vi "task2.vi"(6 "Zatrzymaj program":bool, 7 "Czy trójkąt jest prostokątny":bool, 8 "Oblicz":bool, 9 "Bok a":dbl(slide)=2.0 scale=0.0..10.0, 10 "Bok b":dbl(slide)=2.0 scale=0.0..10.0, 11 "Bok c":dbl(slide)=2.0 scale=0.0..10.0) -> (1 "Trójkąt:":string, 2 "Obwód trójkąta":dbl, 3 "Pole trójkąta":dbl)   [LabVIEW 2021]
doc: "Aplikacja na bazie maszyny stanów, która liczy pole i obwód podanego trójkąta. Użyty jest w nim program z wcześniejszego zadania. Program sprawdza czy podany trójkąt jest trójkątem prostokątnym."
panel:
  # "Podaj wielkość trójkąta:"
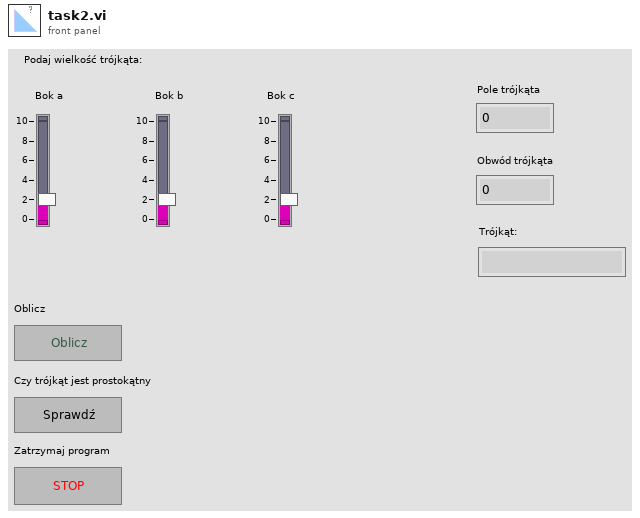
[diagram p1: front panel]
types:
  T1 = enum16{"Idle", "Czy prostokątny", "Oblicz", "Stop"}
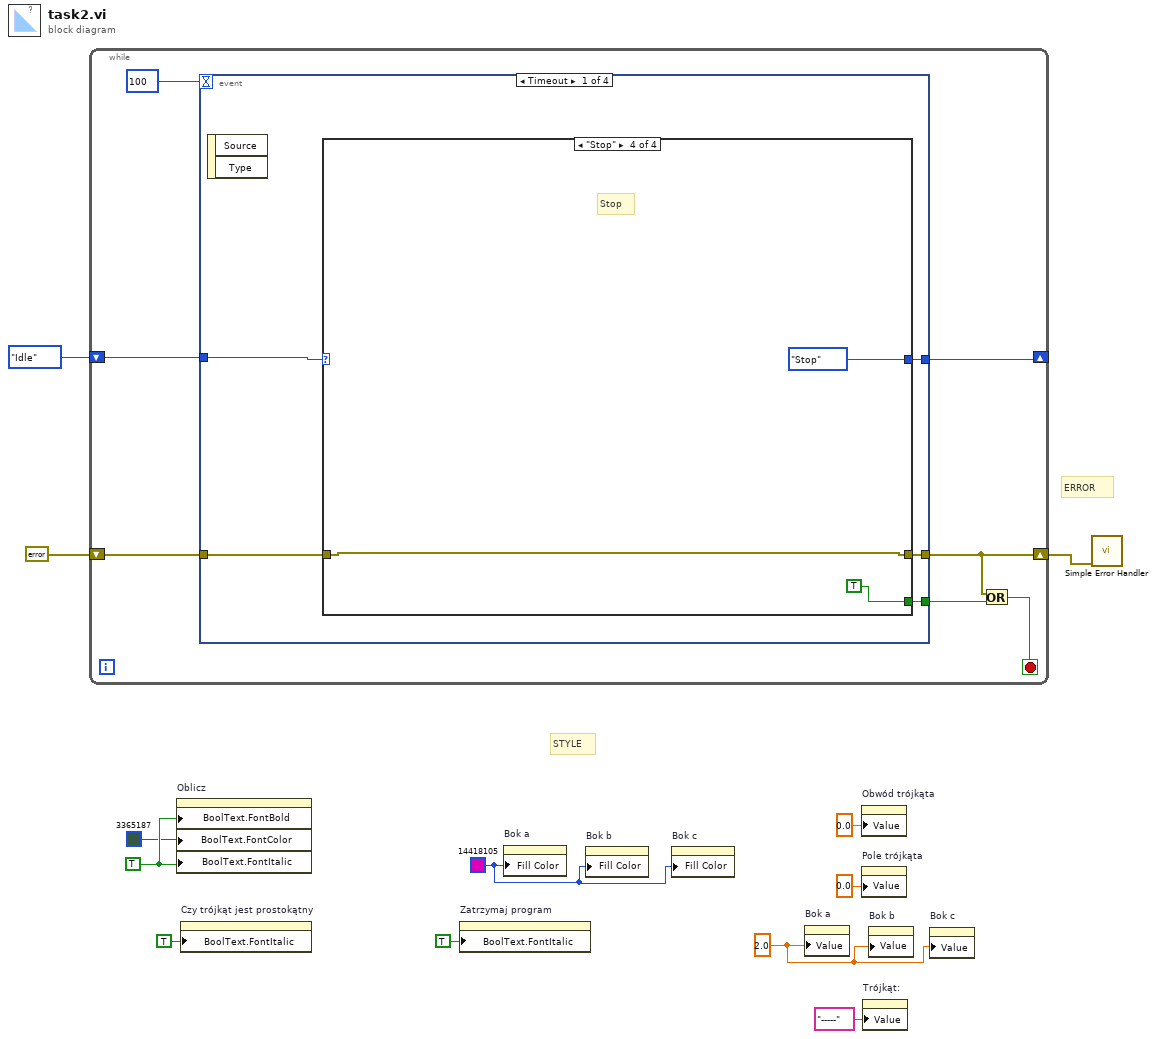
[diagram p0: block diagram]
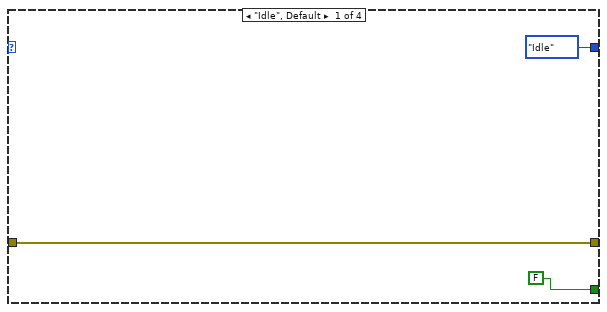
[diagram p2: hidden frame]
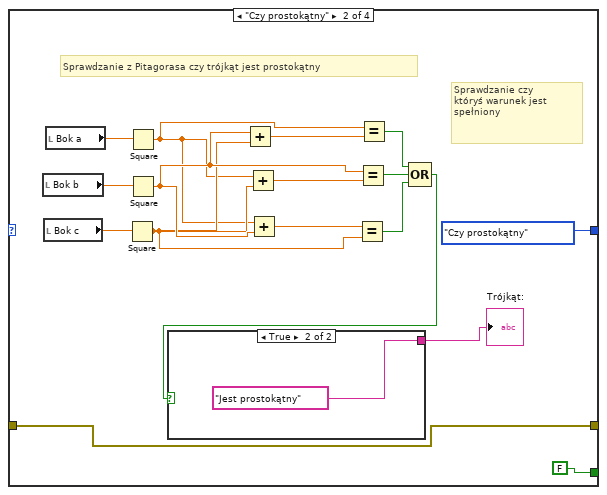
[diagram p3: hidden frame]
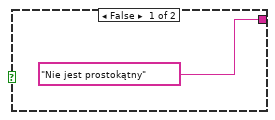
[diagram p4: hidden frame]
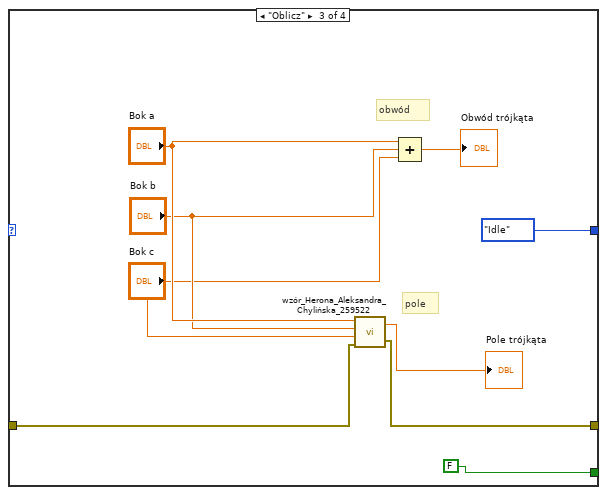
[diagram p5: hidden frame]
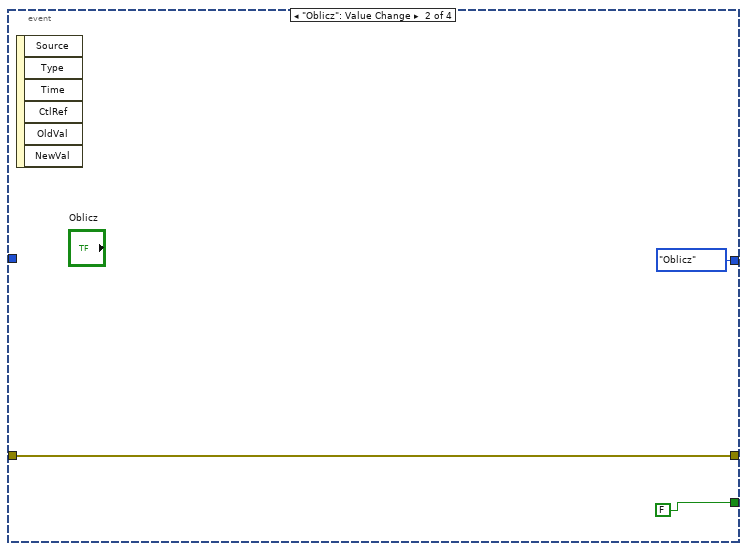
[diagram p6: hidden frame]
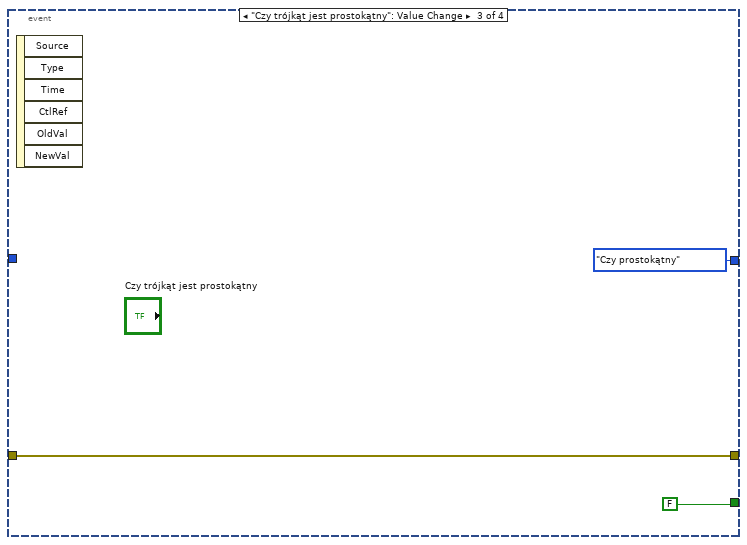
[diagram p7: hidden frame]
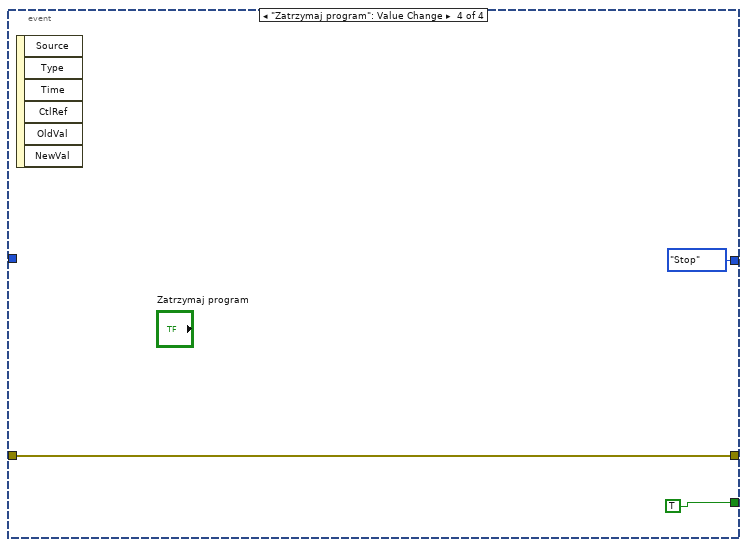
[diagram p8: hidden frame]
diagram:
  w4 = 2.0 ("Bok a")
  w8 = TRUE ("Boolean Text.Font:Italic")
  w9 = u32 14418105 ("Fill Color")
  # "ERROR"
  # "STYLE"
  n1 = while {
    shift-right: [w18] -> _
    shift-left: T1."Idle" -> [w19]
    shift-right: [w14] -> w10
    shift-left: errorcluster {"status"=FALSE, "code"=0, "source"=""} ("error in (no error)") -> [w16]
    stop <- w15 stop-if-true
    n2 = event shown="[0] Timeout" {
      selector: _ -> [_ _ _ _]
      dyn-events: _ -> [_ _ _ _]
      timeout: 100 -> [_ _ _ _]
      tunnel: w19 -> [w24 _ _ _]
      tunnel: [w23 T1."Oblicz" T1."Czy prostokątny" T1."Stop"] -> w18
      tunnel: w16 -> [w22 w60 w63 w66]
      tunnel: [w21 w60 w63 w66] -> w14
      tunnel: [w20 FALSE FALSE TRUE] -> w13
      event Timeout {
        n3 = event-data() -> ()  [unwired: 1 in, 2 out]
        n4 = case shown="\"Stop\"" w24 {
          tunnel: [T1."Idle" T1."Czy prostokątny" T1."Idle" T1."Stop"] -> w23
          tunnel: w22 -> [w26 w29 w49 w57]
          tunnel: [w26 w29 w48 w57] -> w21
          tunnel: [FALSE FALSE FALSE TRUE] -> w20
          frame "Idle", Default {
          }
          frame "Czy prostokątny" {
            # "Sprawdzanie z Pitagorasa czy trójkąt jest prostokątny"
            # "Sprawdzanie czy\nktóryś warunek jest\nspełniony"
            n5 = local read "Bok b"() -> (w42:dbl)
            n6 = local read "Bok c"() -> (w41:dbl)
            n7 = local read "Bok a"() -> (w43:dbl)
            n8 = Square(x=w41) -> (x^2=w37:dbl)
            n9 = Square(x=w43) -> (x^2=w35:dbl)
            n10 = Square(x=w42) -> (x^2=w38:dbl)
            n11 = Add(x=w38, y=w37) -> (x+y=w40:dbl)
            n12 = Add(x=w35, y=w37) -> (x+y=w39:dbl)
            n13 = Add(x=w35, y=w38) -> (x+y=w36:dbl)
            n14 = Equal?(x=w36, y=w37) -> (x = y?=w31:bool)
            n15 = Equal?(x=w38, y=w39) -> (x = y?=w32:bool)
            n16 = Equal?(x=w35, y=w40) -> (x = y?=w33:bool)
            n17 = Compound Arithmetic op=OR(w33, w32, w31) -> (w34:bool)
            n18 = case shown="True" w34 {
              tunnel: ["Nie jest prostokątny" "Jest prostokątny"] -> w30
              frame False {
              }
              frame True {
              }
            }
            "Trójkąt:" <- w30
          }
          frame "Oblicz" {
            # "pole"
            # "obwód"
            n19 = call "wzór_Herona_Aleksandra_Chylińska_259522.vi"("error in (no error)"=w49, "c"="Bok c", "b"="Bok b", "a"="Bok a") -> ("error out"=w48:errorcluster, "Pole trójkąta"=→"Pole trójkąta":dbl)
            n20 = Compound Arithmetic op=ADD("Bok a", "Bok b", "Bok c") -> (→"Obwód trójkąta":dbl)
          }
          frame "Stop" {
            # "Stop"
          }
        }
      }
      event "Oblicz": Value Change {
        n21 = event-data() -> ()  [unwired: 1 in, 6 out]
      }
      event "Czy trójkąt jest prostokątny": Value Change {
        n22 = event-data() -> ()  [unwired: 1 in, 6 out]
      }
      event "Zatrzymaj program": Value Change {
        n23 = event-data() -> ()  [unwired: 1 in, 6 out]
      }
    }
    n24 = Or(x=w14, y=w13) -> (x .or. y?=w15:bool)
  }
  n25 = property on="Oblicz" class="Bool"("BoolText.FontBold"=w8, "BoolText.FontColor"=u32 3365187 ("Boolean Text.Font:Color"), "BoolText.FontItalic"=w8) -> ()  [unwired: 2 in, 2 out]
  n26 = property on="Czy trójkąt jest prostokątny" class="Bool"("BoolText.FontItalic"=TRUE ("Boolean Text.Font:Italic")) -> ()  [unwired: 2 in, 2 out]
  n27 = property on="Zatrzymaj program" class="Bool"("BoolText.FontItalic"=TRUE ("Boolean Text.Font:Italic")) -> ()  [unwired: 2 in, 2 out]
  n28 = property on="Bok a" class="Slide (strict)"("Fill Color"=w9) -> ()  [unwired: 2 in, 2 out]
  n29 = property on="Bok b" class="Slide (strict)"("Fill Color"=w9) -> ()  [unwired: 2 in, 2 out]
  n30 = property on="Bok c" class="Slide (strict)"("Fill Color"=w9) -> ()  [unwired: 2 in, 2 out]
  n31 = property on="Bok a" class="Slide (strict)"("Value"=w4) -> ()  [unwired: 2 in, 2 out]
  n32 = property on="Obwód trójkąta" class="DigNum (strict)"("Value"=0.0 ("Obwód trójkąta")) -> ()  [unwired: 2 in, 2 out]
  n33 = property on="Pole trójkąta" class="DigNum (strict)"("Value"=0.0 ("Pole trójkąta")) -> ()  [unwired: 2 in, 2 out]
  n34 = property on="Trójkąt:" class="Str"("Value"="-----" ("Trójkąt:")) -> ()  [unwired: 2 in, 2 out]
  n35 = property on="Bok b" class="Slide (strict)"("Value"=w4) -> ()  [unwired: 2 in, 2 out]
  n36 = property on="Bok c" class="Slide (strict)"("Value"=w4) -> ()  [unwired: 2 in, 2 out]
  n37 = call <vilib>:"Simple Error Handler.vi"("error in (no error)"=w10) -> ()  [unwired: 4 in, 5 out]
